vi "HOST_GIPO.vi"() -> ()   [LabVIEW 2018]
uses:
  Program Files (x86)/National Instruments/LabVIEW 2018/examples/Instrument IO/Serial/support/Serial - Settings.ctl
  <instrlib>/niDCPower/nidcpower.llb/niDCPower Measurement Type.ctl
  <vilib>/Instr/_visa.llb/VISA Configure Serial Port (Instr).vi
panel:
  out "CPTE_0":bool
  in  "Запись":bool
  in  "Инициализация":string[](array[string])=["QUITE 0", "INT 0", "OUTP 0", "PAR 0", "PAR:DEL 0", "CH:1:THR 50", "CH:2:THR 50", "CH:3:THR 50", "CH:4:THR 50"]
  in  "Команды":string="INT [1,0,?] - Enabled/Disabled/Get Interrupt\nQUITE [1,0,?] - Enabled/Disabled/Get QuiteMode\nOUTP [1,0,?] - On/Off/Get Output\nRESU - Block parry, on output and unblock parry\nRESU:DEL - Delay in ms of block parry\nRESU:AUTO [1,0,?] - Auto resume after parry\nRESU:AUTO:DEL - Delay in ms of Auto resume\nMON [1,0,?] - Enabled/Disabled/Get Monitor\nMON:DEL [0-1000,?] - Set/Get Monitor Delay in ms of Monitor\nPAR [1,0,?] - Enabled/Disabled/Get Parry\nPAR:DEL [0-1000,?] - Set/Get Parry Delay in ms of Parry\nCH:i:MEAS:CURR? - Measure current in channel [i]\nCH:i:MAX:CURR? - Get max current in channel [i], and clear value\nCH:i:THR [20-3330,?] - Set/Get Threshold current in mA in channel [i] of SEL Event\nCH:i:STAT? - Get State of channel [i]\nUse number 0 for alternate channel, and Threshold from [1-1666] mA\nCHSSTAT? - Get State channels\nCHSEXST? - Get Exist channels\nCNT? - Get count SEL\nCNT:CLR - Clear count SEL\nWIRECLOCK [100000,400000] - set I2C clock\nTEST - Self test ADC + DAC + Triggers"
  in  "Ручной(Т)/Авто":bool
  in  "Log":string="Ниже представлен лог общения с СПТЭ:\nParry Scheme initialized.v2.9.2 + Alt Channel\nSend <HELP> to see commands.\nNow set Ipar = 333 mA (Upar = 0.5 V, Upar_alt = 3.0 V)\nExist channels\nCh1 : 1\nCh2 : 1\nCh3 : 1\nCh4 : 1\nCh_alt0 : 0\nREADY\nQUITE Off\nINT Off\nOUTP Off\nPAR Off\nPAR:DEL: 0 ms\nIn ch1 (DAC 0xC) set Ipar = 20 mA (0.030 V)\nIn ch2 (DAC 0xD) set Ipar = 20 mA (0.030 V)\nIn ch3 (DAC 0xE) set Ipar = 20 mA (0.030 V)\nIn ch4 (DAC 0x8) set Ipar = 20 mA (0.030 V)\ninvalid String, send <HELP> for see commands\nDEBUG:ttyData=\nlength=0\n0x00 0x00 0x00 0x00 0x00 0x00 \n"
  out "CPTE":i32
  out "CPTE":bool
  out "CPTE =":string
  in  "Опрос":bool
  in  "Питание матрицы":bool
  in  "Emt(T)/Enter(F)":bool
  out "Номер образца":string="0"
  in  "SEL":path=path "C:/LabView_PRJ/22.099_GIPO/SEL"
  in  "V_2/GIPO":refnum<k15>="PXI1Slot4" caption="instrument handle"
  in  "V_18/V_65":refnum<k15>="PXI1Slot3" caption="instrument handle"
  in  "V_5/V_55":refnum<k15>="PXI1Slot2" caption="instrument handle"
  out "GIPO Chart":dbl(graph)=0.0015269744355577005 caption="Waveform Chart 5"
  out "GIPO_cur, A":dbl caption="measurement" format="%_6g"
  in  "GIPO_curlim, A":dbl=1.0 caption="current limit" format="%_6p"
  in  "GIPO, V":dbl=16.0 caption="voltage level" format="%_6p"
  out "V_2 Chart":dbl(graph)=0.012083984740959104 caption="Waveform Chart 5"
  out "V_2_cur, A":dbl caption="measurement" format="%_6g"
  in  "V_2_curlim, A":dbl=0.1 caption="current limit" format="%_6p"
  in  "V_2, V":dbl=2.048 caption="voltage level" format="%_6p"
  in  "Питание":bool
  out "V_65 Chart":dbl(graph)=0.002248520443690256
  out "V_65_cur, A":dbl caption="measurement" format="%_6g"
  in  "V_65, V":dbl=6.5 caption="voltage level" format="%_6p"
  in  "V_65_curlim, A":dbl=0.1 caption="current limit" format="%_6p"
  out "V_5 Chart":dbl(graph)=0.10501062604189042 caption="Waveform Chart 5"
  out "V_18 Chart":dbl(graph)=0.06950688300254347
  out "V_55 Chart":dbl(graph)=0.0003386853255381902
  out "V_18_cur, A":dbl caption="measurement" format="%_6g"
  in  "V_18_curlim, A":dbl=0.1 caption="current limit" format="%_6p"
  in  "V_18, V":dbl=1.8 caption="voltage level" format="%_6p"
  in  "V_55, V":dbl=5.5 caption="voltage level" format="%_6p"
  out "V_55_cur, A":dbl caption="measurement" format="%_6g"
  out "V_5_cur, A":dbl caption="measurement" format="%_6g"
  in  "V_55_curlim, A":dbl=0.1 caption="current limit" format="%_6p"
  in  "V_5_curlim, A":dbl=0.1 caption="current limit" format="%_6p"
  in  "V_5, V":dbl=5.0 caption="voltage level" format="%_6p"
  in  "Стоп":bool
  in  "Период, мс":u32=1
  out "V_2":bool
  out "V_2":i32
  in  "V_2_selcur":dbl=0.01 caption="current limit" format="%_6p"
  out "V_65":bool
  out "V_65":i32
  in  "V_65_selcur":dbl=0.01 caption="current limit" format="%_6p"
  out "V_18":bool
  out "V_18":i32
  out "V_55":bool
  out "V_55":i32
  out "V_5":bool
  out "V_5":i32
  in  "V_18_selcur":dbl=0.01 caption="current limit" format="%_6p"
  in  "V_55_selcur":dbl=0.01 caption="current limit" format="%_6p"
  in  "V_5_selcur":dbl=0.01 caption="current limit" format="%_6p"
  out "SEL":bool
  in  "SIM_SEL":bool
  out "GIPO":bool
  out "GIPO":i32
  in  "GIPO_selcur":dbl=0.95 caption="current limit" format="%_6p"
  in  "Питание оснастки":bool
  in  "Command":string="PAR 0"
  in  "Serial Settings":T1={"baud rate"=115200, "data bits"=8, "parity"=enum."None", "stop bits"=10, "flow control"=0} {"flow control" items=["None"=0, "XON/XOFF"=1, "RTS/CTS"=2, "DTR/DSR"=4]; "stop bits" items=["1.0"=10, "1.5"=15, "2.0"=20]; "data bits" min=5 max=8 step=1; "baud rate" items=["75"=75, "110"=110, "134"=134, "150"=150, "300"=300, "600"=600, "1200"=1200, "1800"=1800, "2400"=2400, "4800"=4800, "7200"=7200, "9600"=9600, "14400"=14400, "19200"=19200, "28800"=28800, "38400"=38400, "56000"=56000, "57600"=57600, "115200"=115200, "128000"=128000, "230400"=230400]}
  in  "VISA resource name":refnum<visa-resource-name>="COM4"
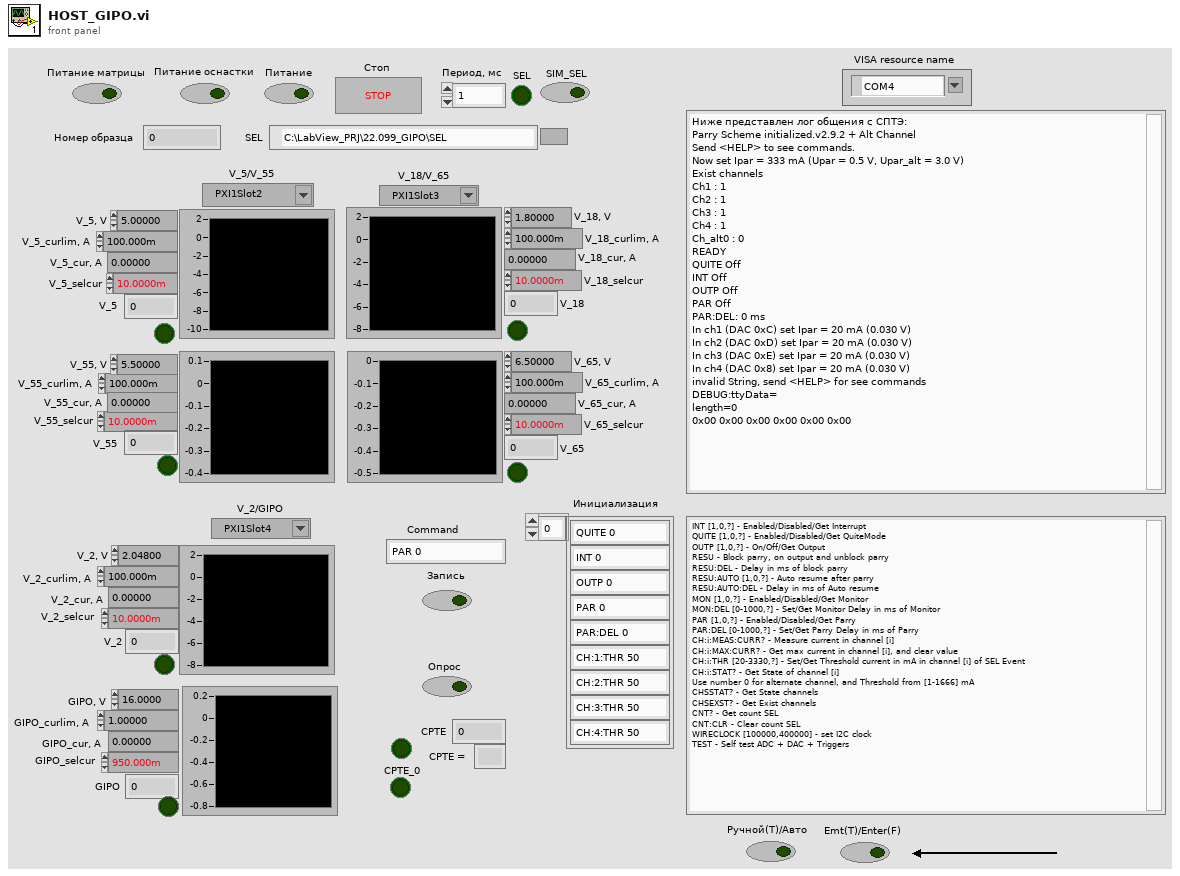
[diagram p1: front panel]
types:
  T1 = typedef "Serial - Settings.ctl" = cluster{"baud rate":u32, "data bits":u16, "parity":enum16{"None", "Odd", "Even", "Mark", "Space"}, "stop bits":u16, "flow control":u16}
  T2 = enum16{"open", "replace", "create", "open or create", "replace or create", "replace or create with confirmation"}
  T3 = enum16{"Native", "Native Command Line", "UNIX", "Macintosh", "DOS"}
  T4 = typedef "niDCPower Measurement Type.ctl" = i32
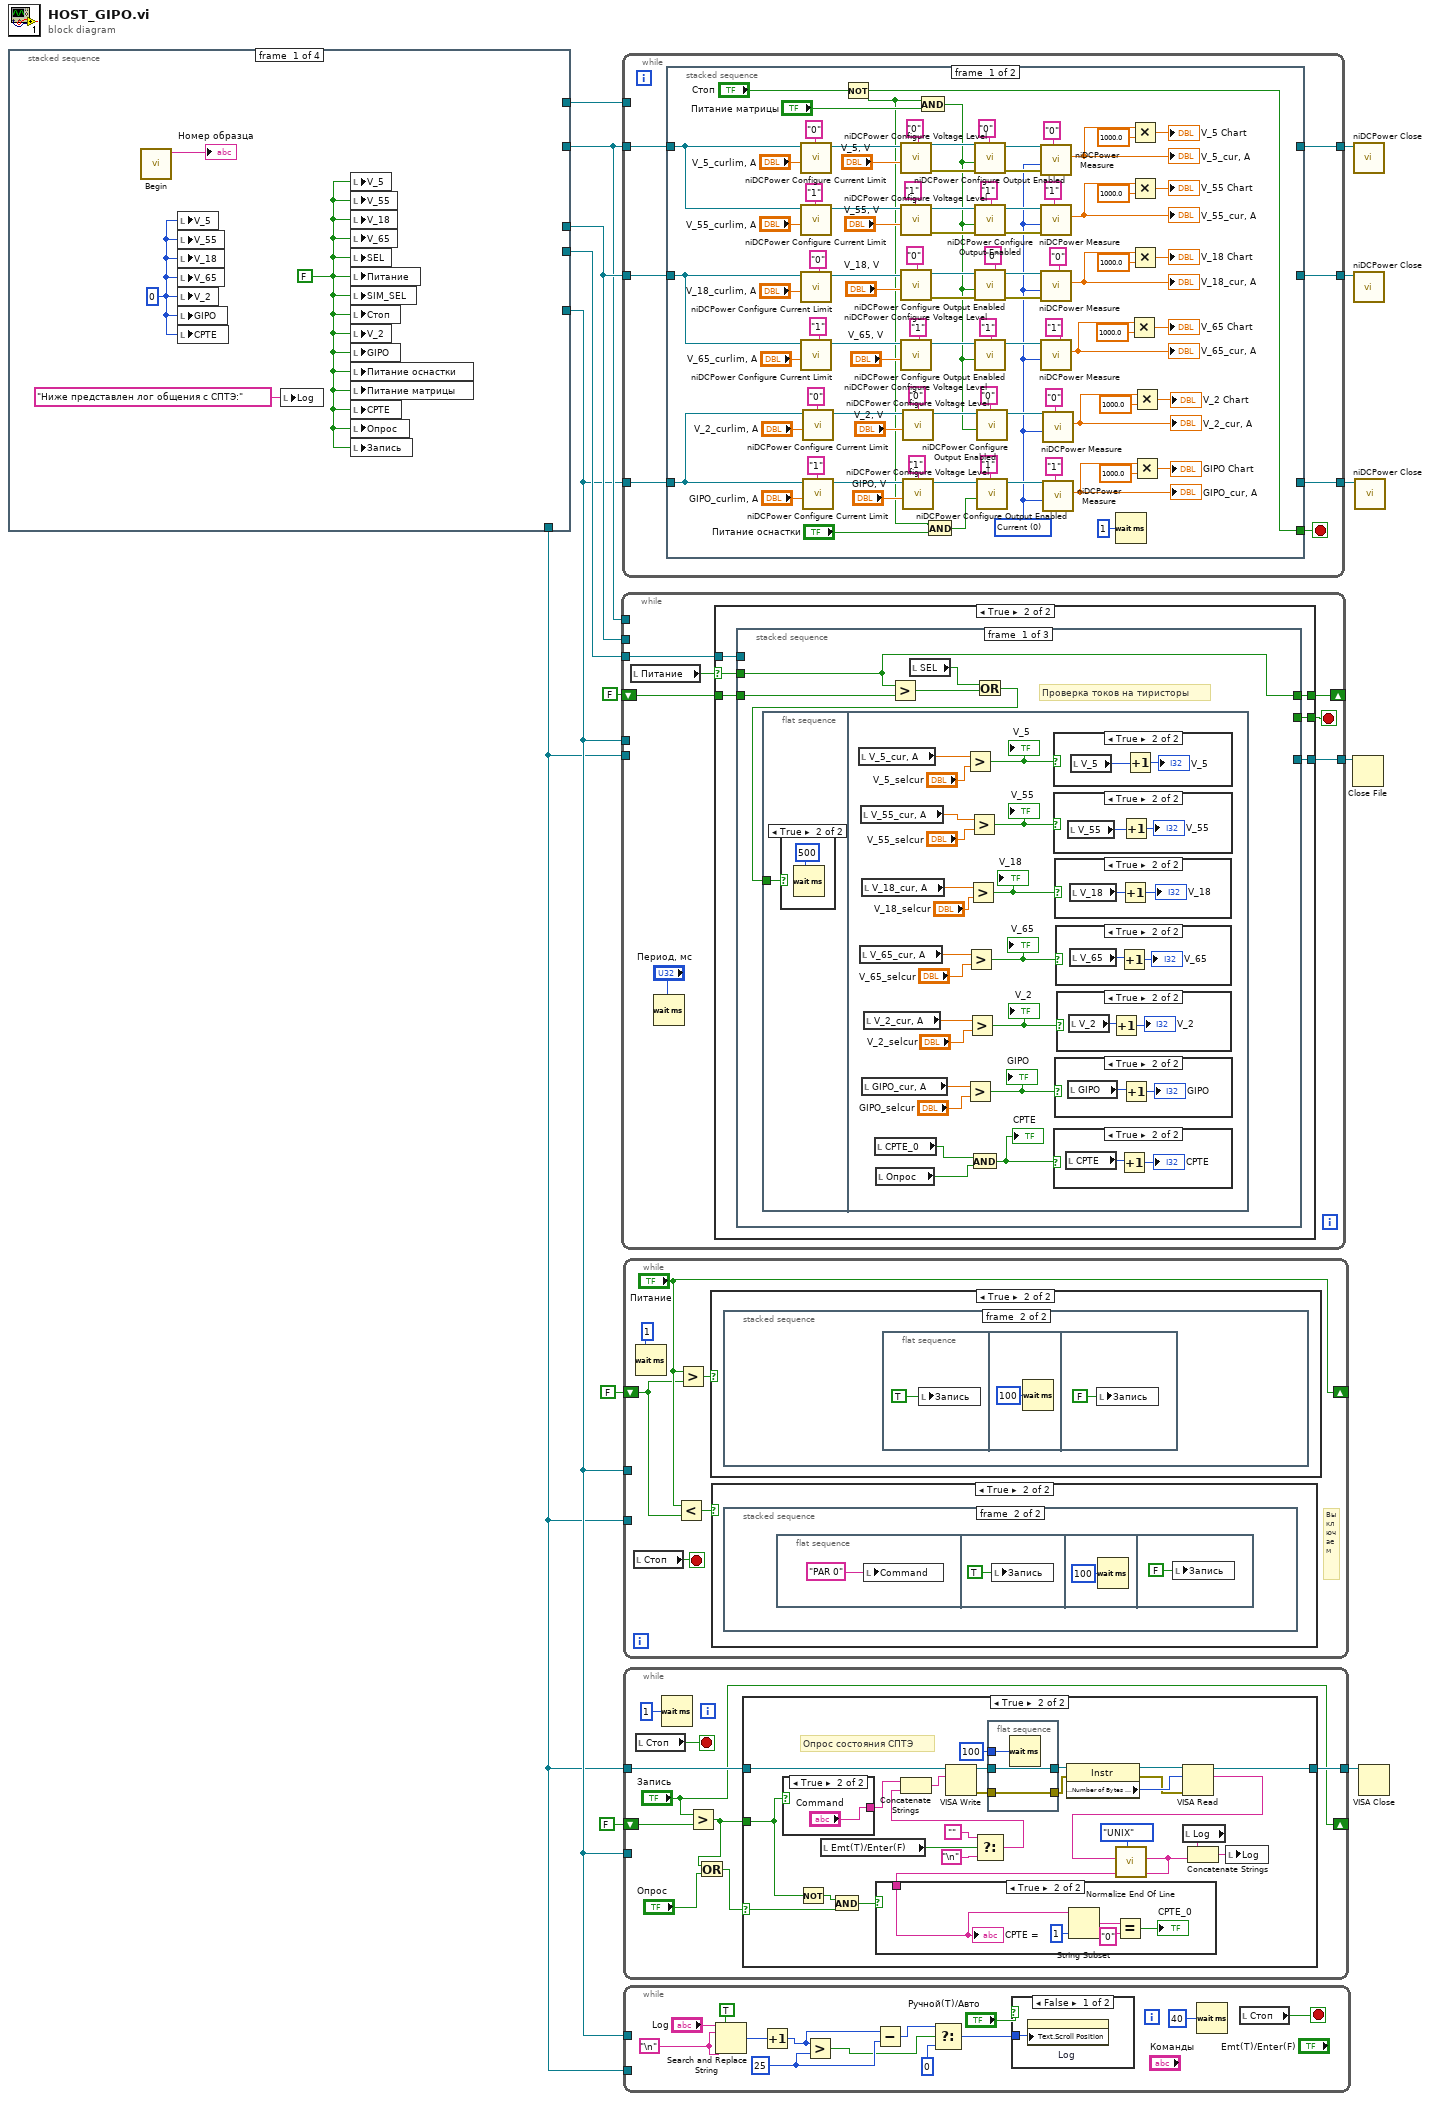
[diagram p0: block diagram]
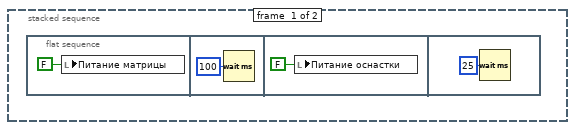
[diagram p3: hidden frame]
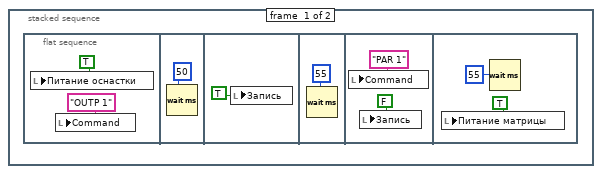
[diagram p5: hidden frame]
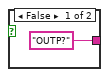
[diagram p8: hidden frame]
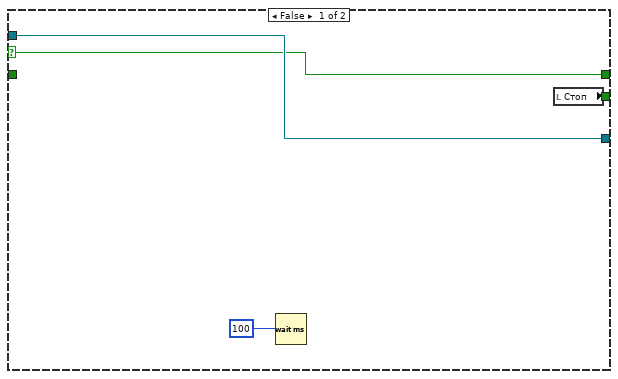
[diagram p10: hidden frame]
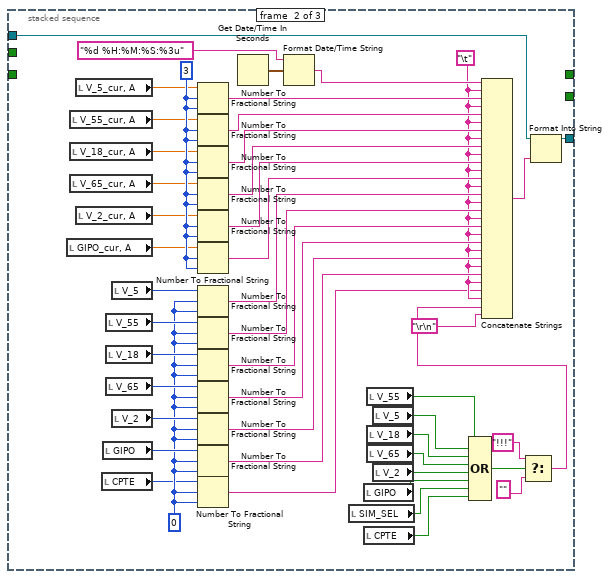
[diagram p19: hidden frame]
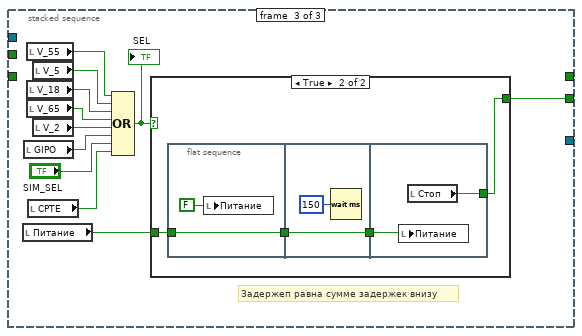
[diagram p20: hidden frame]
diagram:
  n1 = stacked-sequence {
    tunnel: [_ _ w67 _] -> w11
    tunnel: [_ _ w66 _] -> w10
    tunnel: [_ w36 _ _] -> w13
    tunnel: [_ _ w60 _] -> w5
    tunnel: [_ _ _ w85] -> w6
    tunnel: [_ _ _ w85] -> w4
    frame #0 {
      w17 = 0
      w16 = FALSE
      n2 = call "Begin.vi"() -> ("Номер образца 2"=→"Номер образца":string)  [unwired: 11 in]
      n3 = local write "V_5"(w17) -> ()
      n4 = local write "V_55"(w17) -> ()
      n5 = local write "V_18"(w17) -> ()
      n6 = local write "V_65"(w17) -> ()
      n7 = local write "V_2"(w17) -> ()
      n8 = local write "GIPO"(w17) -> ()
      n9 = local write "CPTE"(w17) -> ()
      n10 = local write "Log"("Ниже представлен лог общения с СПТЭ:") -> ()
      n11 = local write "V_5"(w16) -> ()
      n12 = local write "V_55"(w16) -> ()
      n13 = local write "V_18"(w16) -> ()
      n14 = local write "V_65"(w16) -> ()
      n15 = local write "SEL"(w16) -> ()
      n16 = local write "Питание"(w16) -> ()
      n17 = local write "SIM_SEL"(w16) -> ()
      n18 = local write "Стоп"(w16) -> ()
      n19 = local write "V_2"(w16) -> ()
      n20 = local write "GIPO"(w16) -> ()
      n21 = local write "Питание оснастки"(w16) -> ()
      n22 = local write "Питание матрицы"(w16) -> ()
      n23 = local write "CPTE"(w16) -> ()
      n24 = local write "Опрос"(w16) -> ()
      n25 = local write "Запись"(w16) -> ()
    }
    frame #1 {
      w21 = "\t"
      # "Инициализаци первой строки лога по токам"
      n26 = local read "Номер образца"() -> (w48:string)
      n27 = Build Path(base path="SEL", name or relative path=w48) -> (appended path=w50:path)
      n28 = Get Date/Time In Seconds() -> (seconds since 1Jan1904=w43:timestamp)
      n29 = call <vilib>:"Check if File or Folder Exists.vi"("path"=w50) -> ("file or folder exists?"=w51:bool, "dup path"=w52:path)  [unwired: 8 in, 1 out]
      n30 = Format Date/Time String(time format string (%c)="%d %H.%M.%S", seconds (now)=w43) -> (date/time string=w40:string)  [unwired: 1 in]
      n31 = case shown="False" w51 {
        tunnel: w52 -> [w58 w59]
        tunnel: [w57 w59] -> w35
        frame False {
          n32 = Create Folder(path (use dialog)=w58) -> (created path=w57:path)  [unwired: 2 in, 2 out]
        }
        frame True {
        }
      }
      n33 = Concatenate Strings(w40, ".xls" ("string")) -> (w38:string)
      n34 = Build Path(base path=w35, name or relative path=w38) -> (appended path=w41:path)
      n35 = Open/Create/Replace File(file path (use dialog)=w41, operation (0:open)=T2."open or create", access (0:read/write)=enum16{"read/write", "read-only", "write-only"}."read/write") -> (refnum out=w44:refnum<file>)  [unwired: 3 in, 2 out]
      n36 = case shown="True" TRUE {
        tunnel: w44 -> [w53 w56]
        tunnel: [w53 w54] -> w37
        frame False {
        }
        frame True {
          n37 = Set File Position(refnum=w56, from (0:start)=enum16{"start", "end", "current"}."end") -> (refnum out=w54:refnum<file>)  [unwired: 2 in, 1 out]
        }
      }
      n38 = Format Into String(initial string=w37, "Time" ("input 1"), w21, "V_5_cur " ("input 1"), w21, "V_55_cur " ("input 1"), w21, "V_18_cur " ("input 1"), w21, "V_65_cur " ("input 1"), w21, "V_2_cur " ("input 1"), w21, "GIPO_cur " ("input 1"), w21, "V_5" ("input 1"), w21, "V_55" ("input 1"), w21, "V_18" ("input 1"), w21, "V_65" ("input 1"), w21, "V_2" ("input 1"), w21, "GIPO" ("input 1"), w21, "CPTE" ("input 1"), "\r\n") -> (resulting string=w36:refnum<file>)  [unwired: 2 in, 1 out]
    }
    frame #2 {
      n39 = call <instrlib>:"niDCPower Initialize.vi"("resource name"="V_2/GIPO") -> ("error out"=w63:errorcluster, "instrument handle out"=w62:refnum<k15>)  [unwired: 3 in, 6 out]
      n40 = call <instrlib>:"niDCPower Initialize.vi"("resource name"="V_5/V_55") -> ("error out"=w74:errorcluster, "instrument handle out"=w76:refnum<k15>)  [unwired: 3 in, 6 out]
      n41 = call <instrlib>:"niDCPower Initialize.vi"("resource name"="V_18/V_65") -> ("error out"=w75:errorcluster, "instrument handle out"=w77:refnum<k15>)  [unwired: 3 in, 6 out]
      n42 = call <instrlib>:"niDCPower Configure Voltage Level.vi"("error in (no error)"=w74, "voltage level"=0.0, "channel name"="0,1", "instrument handle"=w76) -> ("instrument handle out"=w66:refnum<k15>)  [unwired: 6 in, 1 out]
      n43 = call <instrlib>:"niDCPower Configure Voltage Level.vi"("error in (no error)"=w75, "voltage level"=0.0, "channel name"="0,1", "instrument handle"=w77) -> ("instrument handle out"=w67:refnum<k15>)  [unwired: 6 in, 1 out]
      n44 = call <instrlib>:"niDCPower Configure Voltage Level.vi"("error in (no error)"=w63, "voltage level"=0.0, "channel name"="0,1", "instrument handle"=w62) -> ("instrument handle out"=w60:refnum<k15>)  [unwired: 6 in, 1 out]
    }
    frame #3 {
      n45 = Unbundle By Name("Serial Settings") -> ("baud rate"=w98:u32, "data bits"=w97:u16, "parity"=w96:enum16{"None", "Odd", "Even", "Mark", "Space"}, "stop bits"=w95:u16, "flow control"=w94:u16)
      n46 = for {
        tunnel: "Инициализация" -> [w108] mode=indexing
        tunnel: w87 -> [w111]
        tunnel: [w109] -> w86
        n47 = local read "Emt(T)/Enter(F)"() -> (w106:bool)
        n48 = Select(t="", s=w106, f="\n") -> (s? t:f=w103:string)
        n49 = Concatenate Strings(w108, w103) -> (w107:string)
        n50 = VISA Write(VISA resource name=w111, write buffer=w107) -> (VISA resource name out=w110:refnum<visa-resource-name>)  [unwired: 1 in, 2 out]
        n51 = flat-sequence {
          tunnel: [w113] -> w109
          tunnel: w110 -> [w113]
          frame #0 {
            n52 = Wait (ms)(milliseconds to wait=u32 100) -> ()  [unwired: 1 out]
          }
        }
      }
      n53 = property class="Instr"(reference=w86) -> (reference out=w91:refnum<visa-resource-name>, error out=w90:errorcluster, "Serial Settings:Number of Bytes at Serial Port"=w89:u32)  [unwired: 1 in]
      n54 = VISA Read(VISA resource name=w91, byte count=w89, error in (no error)=w90) -> (VISA resource name out=w85:refnum<visa-resource-name>, read buffer=w83:string)  [unwired: 2 out]
      n55 = call-poly "VISA Configure Serial Port"("VISA resource name"="VISA resource name", "termination char\n(0xA = '\\n' = LF)"=u8 10 ("termination char\n(0xA = '\\n' = LF)"), "Enable Termination\nChar (T)"=FALSE ("Enable Termination\nChar (T)"), "baud rate (9600)"=w98, "data bits (8)"=w97, "parity (0:none)"=w96, "stop bits (10: 1 bit)"=w95, "flow control (0:none)"=w94) -> ("VISA resource name out"=w88:refnum<visa-resource-name>)  [unwired: 2 in, 5 out]
      n56 = call <vilib>:"Normalize End Of Line.vi"("end of line (Native)"=T3."UNIX", "string in"=w83) -> ("string out"=w82:string)  [unwired: 6 in]
      n57 = flat-sequence {
        tunnel: w88 -> [w101]
        tunnel: [w101] -> w87
        frame #0 {
          n58 = Wait (ms)(milliseconds to wait=u32 2000) -> ()  [unwired: 1 out]
        }
      }
      n59 = local read "Log"() -> (w80:string)
      n60 = Concatenate Strings(w80, "\n", w82) -> (w84:string)
      n61 = local write "Log"(w84) -> ()
    }
  }
  n62 = while {
    shift-right: [w114] -> _
    shift-left: FALSE -> [w120]
    tunnel: w13 -> [w119]
    tunnel: [w117] -> w12
    tunnel: w5 -> [_]
    tunnel: w11 -> [_]
    tunnel: w10 -> [_]
    tunnel: w4 -> [_]
    stop <- w118 stop-if-true
    n63 = local read "Питание"() -> (w115:bool)
    n64 = Wait (ms)(milliseconds to wait="Период, мс") -> ()  [unwired: 1 out]
    n65 = case shown="True" w115 {
      selector: w115 -> [w121 w126]
      tunnel: w120 -> [_ w130]
      tunnel: w119 -> [w123 w129]
      tunnel: [w124 w128] -> w118
      tunnel: [w123 w127] -> w117
      tunnel: [w121 w125] -> w114
      frame False {
        n66 = Wait (ms)(milliseconds to wait=u32 100 ("f")) -> ()  [unwired: 1 out]
        n67 = local read "Стоп"() -> (w124:bool)
      }
      frame True {
        n68 = stacked-sequence {
          tunnel: w130 -> [w135 _ _]
          tunnel: w129 -> [_ w210 _]
          tunnel: [_ _ w222] -> w128
          tunnel: [_ w208 _] -> w127
          tunnel: w126 -> [w131 _ _]
          tunnel: [w131 _ _] -> w125
          frame #0 {
            # "Проверка токов на тиристоры"
            n69 = flat-sequence {
              tunnel: w132 -> [w136]
              frame #0 {
                n70 = case shown="True" w136 {
                  frame False {
                  }
                  frame True {
                    n71 = Wait (ms)(milliseconds to wait=u32 500) -> ()  [unwired: 1 out]
                  }
                }
              }
              frame #1 {
                n72 = local read "V_5_cur, A"() -> (w152:dbl)
                n73 = local read "V_65_cur, A"() -> (w149:dbl)
                n74 = local read "V_55_cur, A"() -> (w151:dbl)
                n75 = local read "V_18_cur, A"() -> (w150:dbl)
                n76 = local read "GIPO_cur, A"() -> (w141:dbl)
                n77 = local read "V_2_cur, A"() -> (w144:dbl)
                n78 = local read "CPTE_0"() -> (w139:bool)
                n79 = local read "Опрос"() -> (w138:bool)
                n80 = Greater?(x=w152, y="V_5_selcur") -> (0:w157:bool)
                "V_5" <- w157
                n81 = Greater?(x=w141, y="GIPO_selcur") -> (0:w143:bool)
                "GIPO" <- w143
                n82 = Greater?(x=w149, y="V_65_selcur") -> (0:w148:bool)
                "V_65" <- w148
                n83 = Greater?(x=w144, y="V_2_selcur") -> (0:w145:bool)
                "V_2" <- w145
                n84 = Greater?(x=w150, y="V_18_selcur") -> (0:w153:bool)
                "V_18" <- w153
                n85 = Greater?(x=w151, y="V_55_selcur") -> (0:w155:bool)
                "V_55" <- w155
                n86 = And(x=w139, y=w138) -> (x .and. y?=w140:bool)
                "CPTE" <- w140
                n87 = case shown="True" w157 {
                  frame False {
                  }
                  frame True {
                    n88 = local read "V_5"() -> (w172:i32)
                    n89 = Increment(x=w172) -> (x+1=→"V_5":i32)
                  }
                }
                n90 = case shown="True" w155 {
                  frame False {
                  }
                  frame True {
                    n91 = local read "V_55"() -> (w169:i32)
                    n92 = Increment(x=w169) -> (x+1=→"V_55":i32)
                  }
                }
                n93 = case shown="True" w140 {
                  frame False {
                  }
                  frame True {
                    n94 = local read "CPTE"() -> (w160:i32)
                    n95 = Increment(x=w160) -> (x+1=→"CPTE":i32)
                  }
                }
                n96 = case shown="True" w153 {
                  frame False {
                  }
                  frame True {
                    n97 = local read "V_18"() -> (w168:i32)
                    n98 = Increment(x=w168) -> (x+1=→"V_18":i32)
                  }
                }
                n99 = case shown="True" w143 {
                  frame False {
                  }
                  frame True {
                    n100 = local read "GIPO"() -> (w162:i32)
                    n101 = Increment(x=w162) -> (x+1=→"GIPO":i32)
                  }
                }
                n102 = case shown="True" w148 {
                  frame False {
                  }
                  frame True {
                    n103 = local read "V_65"() -> (w166:i32)
                    n104 = Increment(x=w166) -> (x+1=→"V_65":i32)
                  }
                }
                n105 = case shown="True" w145 {
                  frame False {
                  }
                  frame True {
                    n106 = local read "V_2"() -> (w164:i32)
                    n107 = Increment(x=w164) -> (x+1=→"V_2":i32)
                  }
                }
              }
            }
            n108 = Greater?(x=w131, y=w135) -> (0:w134:bool)
            n109 = local read "SEL"() -> (w133:bool)
            n110 = Or(x=w133, y=w134) -> (x .or. y?=w132:bool)
          }
          frame #1 {
            w178 = i16 0 ("width (-)")
            w207 = i16 3 ("width (-)")
            w179 = "\t"
            n111 = local read "GIPO_cur, A"() -> (w198:dbl)
            n112 = local read "V_55_cur, A"() -> (w202:dbl)
            n113 = local read "V_18_cur, A"() -> (w201:dbl)
            n114 = local read "V_65_cur, A"() -> (w200:dbl)
            n115 = local read "V_5_cur, A"() -> (w203:dbl)
            n116 = local read "V_2_cur, A"() -> (w199:dbl)
            n117 = local read "CPTE"() -> (w177:i32)
            n118 = local read "GIPO"() -> (w188:i32)
            n119 = local read "V_55"() -> (w196:i32)
            n120 = local read "V_18"() -> (w195:i32)
            n121 = local read "V_65"() -> (w194:i32)
            n122 = local read "V_5"() -> (w197:i32)
            n123 = local read "V_2"() -> (w193:i32)
            n124 = Number To Fractional String(number=w203, width (-)=w207, precision (6)=w207) -> (F-format string=w214:string)  [unwired: 1 in]
            n125 = Number To Fractional String(number=w202, width (-)=w207, precision (6)=w207) -> (F-format string=w213:string)  [unwired: 1 in]
            n126 = Number To Fractional String(number=w201, width (-)=w207, precision (6)=w207) -> (F-format string=w212:string)  [unwired: 1 in]
            n127 = Number To Fractional String(number=w200, width (-)=w207, precision (6)=w207) -> (F-format string=w209:string)  [unwired: 1 in]
            n128 = Number To Fractional String(number=w199, width (-)=w207, precision (6)=w207) -> (F-format string=w205:string)  [unwired: 1 in]
            n129 = Number To Fractional String(number=w198, width (-)=w207, precision (6)=w207) -> (F-format string=w204:string)  [unwired: 1 in]
            n130 = Number To Fractional String(number=w197, width (-)=w178, precision (6)=w178) -> (F-format string=w185:string)  [unwired: 1 in]
            n131 = Number To Fractional String(number=w196, width (-)=w178, precision (6)=w178) -> (F-format string=w184:string)  [unwired: 1 in]
            n132 = Number To Fractional String(number=w195, width (-)=w178, precision (6)=w178) -> (F-format string=w183:string)  [unwired: 1 in]
            n133 = Number To Fractional String(number=w194, width (-)=w178, precision (6)=w178) -> (F-format string=w182:string)  [unwired: 1 in]
            n134 = Number To Fractional String(number=w193, width (-)=w178, precision (6)=w178) -> (F-format string=w181:string)  [unwired: 1 in]
            n135 = Number To Fractional String(number=w188, width (-)=w178, precision (6)=w178) -> (F-format string=w180:string)  [unwired: 1 in]
            n136 = Number To Fractional String(number=w177, width (-)=w178, precision (6)=w178) -> (F-format string=w176:string)  [unwired: 1 in]
            n137 = Get Date/Time In Seconds() -> (seconds since 1Jan1904=w220:timestamp)
            n138 = Format Date/Time String(time format string (%c)="%d %H:%M:%S:%3u", seconds (now)=w220) -> (date/time string=w215:string)  [unwired: 1 in]
            n139 = local read "SIM_SEL"() -> (w186:bool)
            n140 = local read "GIPO"() -> (w187:bool)
            n141 = local read "CPTE"() -> (w173:bool)
            n142 = local read "V_55"() -> (w192:bool)
            n143 = local read "V_18"() -> (w190:bool)
            n144 = local read "V_65"() -> (w189:bool)
            n145 = local read "V_5"() -> (w191:bool)
            n146 = local read "V_2"() -> (w206:bool)
            n147 = Compound Arithmetic op=OR(w192, w191, w190, w189, w206, w187, w186, w173) -> (w211:bool)
            n148 = Select(t="!!!", s=w211, f="") -> (s? t:f=w175:string)
            n149 = Concatenate Strings(w215, w179, w214, w179, w213, w179, w212, w179, w209, w179, w205, w179, w204, w179, w185, w179, w184, w179, w183, w179, w182, w179, w181, w179, w180, w179, w176, w179, w175, "\r\n") -> (w219:string)
            n150 = Format Into String(initial string=w210, w219) -> (resulting string=w208:refnum<file>)  [unwired: 2 in, 1 out]
          }
          frame #2 {
            # "Задержеп равна сумме задержек внизу"
            n151 = local read "Питание"() -> (w221:bool)
            n152 = local read "GIPO"() -> (w225:bool)
            n153 = local read "V_55"() -> (w229:bool)
            n154 = local read "V_18"() -> (w227:bool)
            n155 = local read "V_65"() -> (w226:bool)
            n156 = local read "CPTE"() -> (w223:bool)
            n157 = local read "V_5"() -> (w228:bool)
            n158 = local read "V_2"() -> (w231:bool)
            n159 = Compound Arithmetic op=OR(w229, w228, w227, w226, w231, w225, "SIM_SEL", w223) -> (w230:bool)
            "SEL" <- w230
            n160 = case shown="True" w230 {
              tunnel: [w232 w233] -> w222
              tunnel: w221 -> [_ w234]
              frame False {
                n161 = local read "Стоп"() -> (w232:bool)
              }
              frame True {
                n162 = flat-sequence {
                  tunnel: [w237] -> w235
                  tunnel: w234 -> [w237]
                  tunnel: [w239] -> w236
                  tunnel: w235 -> [w239]
                  tunnel: w236 -> [w242]
                  tunnel: [w241] -> w233
                  frame #0 {
                    n163 = local write "Питание"(FALSE ("Питание")) -> ()
                  }
                  frame #1 {
                    n164 = Wait (ms)(milliseconds to wait=u32 150) -> ()  [unwired: 1 out]
                  }
                  frame #2 {
                    n165 = local write "Питание"(w242) -> ()
                    n166 = local read "Стоп"() -> (w241:bool)
                  }
                }
              }
            }
          }
        }
      }
    }
  }
  n167 = while {
    tunnel: w10 -> [w249]
    tunnel: w5 -> [w247]
    tunnel: w11 -> [w248]
    tunnel: [w246] -> w9
    tunnel: [w245] -> w8
    tunnel: [w244] -> w7
    tunnel: w6 -> [_]
    stop <- w243 stop-if-true
    n168 = stacked-sequence {
      tunnel: w247 -> [w258 w339]
      tunnel: w248 -> [w257 w340]
      tunnel: w249 -> [w256 w341]
      tunnel: [_ w341] -> w246
      tunnel: [_ w340] -> w245
      tunnel: [_ w339] -> w244
      tunnel: ["Стоп" _] -> w243
      frame #0 {
        w259 = T4 0 items=["Current", "Voltage"] ("measurement type")
        n169 = call <instrlib>:"niDCPower Configure Current Limit.vi"("current limit"="V_5_curlim, A", "channel name"="0", "instrument handle"=w256) -> ("instrument handle out"=w327:refnum<k15>)  [unwired: 7 in, 1 out]
        n170 = call <instrlib>:"niDCPower Configure Current Limit.vi"("current limit"="V_55_curlim, A", "channel name"="1", "instrument handle"=w256) -> ("instrument handle out"=w328:refnum<k15>)  [unwired: 7 in, 1 out]
        n171 = call <instrlib>:"niDCPower Configure Current Limit.vi"("current limit"="V_18_curlim, A", "channel name"="0", "instrument handle"=w257) -> ("instrument handle out"=w310:refnum<k15>)  [unwired: 7 in, 1 out]
        n172 = call <instrlib>:"niDCPower Configure Current Limit.vi"("current limit"="V_65_curlim, A", "channel name"="1", "instrument handle"=w257) -> ("instrument handle out"=w290:refnum<k15>)  [unwired: 7 in, 1 out]
        n173 = call <instrlib>:"niDCPower Configure Current Limit.vi"("current limit"="V_2_curlim, A", "channel name"="0", "instrument handle"=w258) -> ("instrument handle out"=w281:refnum<k15>)  [unwired: 7 in, 1 out]
        n174 = call <instrlib>:"niDCPower Configure Current Limit.vi"("current limit"="GIPO_curlim, A", "channel name"="1", "instrument handle"=w258) -> ("instrument handle out"=w262:refnum<k15>)  [unwired: 7 in, 1 out]
        n175 = Not(x="Стоп") -> (.not. x?=w250:bool)
        n176 = call <instrlib>:"niDCPower Configure Voltage Level.vi"("voltage level"="V_5, V", "channel name"="0", "instrument handle"=w327) -> ("error out"=w320:errorcluster, "instrument handle out"=w323:refnum<k15>)  [unwired: 7 in]
        n177 = call <instrlib>:"niDCPower Configure Voltage Level.vi"("voltage level"="V_55, V", "channel name"="1", "instrument handle"=w328) -> ("error out"=w321:errorcluster, "instrument handle out"=w322:refnum<k15>)  [unwired: 7 in]
        n178 = call <instrlib>:"niDCPower Configure Voltage Level.vi"("voltage level"="V_18, V", "channel name"="0", "instrument handle"=w310) -> ("error out"=w314:errorcluster, "instrument handle out"=w315:refnum<k15>)  [unwired: 7 in]
        n179 = call <instrlib>:"niDCPower Configure Voltage Level.vi"("voltage level"="V_65, V", "channel name"="1", "instrument handle"=w290) -> ("instrument handle out"=w288:refnum<k15>)  [unwired: 7 in, 1 out]
        n180 = call <instrlib>:"niDCPower Configure Voltage Level.vi"("voltage level"="V_2, V", "channel name"="0", "instrument handle"=w281) -> ("instrument handle out"=w280:refnum<k15>)  [unwired: 7 in, 1 out]
        n181 = call <instrlib>:"niDCPower Configure Voltage Level.vi"("voltage level"="GIPO, V", "channel name"="1", "instrument handle"=w262) -> ("instrument handle out"=w263:refnum<k15>)  [unwired: 7 in, 1 out]
        n182 = And(x=w250, y="Питание матрицы") -> (x .and. y?=w255:bool)
        n183 = And(x=w250, y="Питание оснастки") -> (x .and. y?=w251:bool)
        n184 = call <instrlib>:"niDCPower Configure Output Enabled.vi"("error in (no error)"=w320, "output enabled"=w255, "channel name"="0", "instrument handle"=w323) -> ("error out"=w332:errorcluster, "instrument handle out"=w331:refnum<k15>)  [unwired: 6 in]
        n185 = call <instrlib>:"niDCPower Configure Output Enabled.vi"("error in (no error)"=w321, "output enabled"=w255, "channel name"="1", "instrument handle"=w322) -> ("error out"=w333:errorcluster, "instrument handle out"=w334:refnum<k15>)  [unwired: 6 in]
        n186 = call <instrlib>:"niDCPower Configure Output Enabled.vi"("error in (no error)"=w314, "output enabled"=w255, "channel name"="0", "instrument handle"=w315) -> ("error out"=w306:errorcluster, "instrument handle out"=w307:refnum<k15>)  [unwired: 6 in]
        n187 = call <instrlib>:"niDCPower Configure Output Enabled.vi"("output enabled"=w255, "channel name"="1", "instrument handle"=w288) -> ("instrument handle out"=w286:refnum<k15>)  [unwired: 7 in, 1 out]
        n188 = call <instrlib>:"niDCPower Configure Output Enabled.vi"("output enabled"=w255, "channel name"="0", "instrument handle"=w280) -> ("instrument handle out"=w279:refnum<k15>)  [unwired: 7 in, 1 out]
        n189 = call <instrlib>:"niDCPower Configure Output Enabled.vi"("output enabled"=w251, "channel name"="1", "instrument handle"=w263) -> ("instrument handle out"=w264:refnum<k15>)  [unwired: 7 in, 1 out]
        n190 = call <instrlib>:"niDCPower Measure.vi"("error in (no error)"=w332, "measurement type"=w259, "channel name"="0", "instrument handle"=w331) -> ("measurement"=w299:dbl)  [unwired: 5 in, 2 out]
        "V_5_cur, A" <- w299
        n191 = call <instrlib>:"niDCPower Measure.vi"("error in (no error)"=w333, "measurement type"=w259, "channel name"="1", "instrument handle"=w334) -> ("measurement"=w302:dbl)  [unwired: 5 in, 2 out]
        "V_55_cur, A" <- w302
        n192 = call <instrlib>:"niDCPower Measure.vi"("error in (no error)"=w306, "measurement type"=w259, "channel name"="0", "instrument handle"=w307) -> ("measurement"=w300:dbl)  [unwired: 5 in, 2 out]
        "V_18_cur, A" <- w300
        n193 = call <instrlib>:"niDCPower Measure.vi"("measurement type"=w259, "channel name"="1", "instrument handle"=w286) -> ("measurement"=w284:dbl)  [unwired: 6 in, 2 out]
        "V_65_cur, A" <- w284
        n194 = call <instrlib>:"niDCPower Measure.vi"("measurement type"=w259, "channel name"="0", "instrument handle"=w279) -> ("measurement"=w278:dbl)  [unwired: 6 in, 2 out]
        "V_2_cur, A" <- w278
        n195 = call <instrlib>:"niDCPower Measure.vi"("measurement type"=w259, "channel name"="1", "instrument handle"=w264) -> ("measurement"=w265:dbl)  [unwired: 6 in, 2 out]
        "GIPO_cur, A" <- w265
        n196 = Wait (ms)(milliseconds to wait=u32 1) -> ()  [unwired: 1 out]
        n197 = Multiply(x=w284, y=1000.0) -> (x*y=→"V_65 Chart":dbl)
        n198 = Multiply(x=w299, y=1000.0) -> (x*y=→"V_5 Chart":dbl)
        n199 = Multiply(x=w302, y=1000.0) -> (x*y=→"V_55 Chart":dbl)
        n200 = Multiply(x=w300, y=1000.0) -> (x*y=→"V_18 Chart":dbl)
        n201 = Multiply(x=w278, y=1000.0) -> (x*y=→"V_2 Chart":dbl)
        n202 = Multiply(x=w265, y=1000.0) -> (x*y=→"GIPO Chart":dbl)
      }
      frame #1 {
      }
    }
  }
  n203 = while {
    tunnel: w5 -> [_]
    tunnel: w4 -> [_]
    shift-right: ["Питание"] -> _
    shift-left: FALSE ("Питание") -> [w344]
    stop <- w347 stop-if-true
    # "Выключаем"
    n204 = local read "Стоп"() -> (w347:bool)
    n205 = Wait (ms)(milliseconds to wait=u32 1) -> ()  [unwired: 1 out]
    n206 = Less?(x="Питание", y=w344) -> (x < y?=w342:bool)
    n207 = Greater?(x="Питание", y=w344) -> (0:w343:bool)
    n208 = case shown="True" w343 {
      frame False {
      }
      frame True {
        n209 = stacked-sequence {
          frame #0 {
            n210 = flat-sequence {
              frame #0 {
                n211 = local write "Питание оснастки"(TRUE ("Питание оснастки")) -> ()
                n212 = local write "Command"("OUTP 1" ("Command")) -> ()
              }
              frame #1 {
                n213 = Wait (ms)(milliseconds to wait=u32 50) -> ()  [unwired: 1 out]
              }
              frame #2 {
                n214 = local write "Запись"(TRUE ("Запись")) -> ()
              }
              frame #3 {
                n215 = Wait (ms)(milliseconds to wait=u32 55) -> ()  [unwired: 1 out]
              }
              frame #4 {
                n216 = local write "Command"("PAR 1" ("Command")) -> ()
                n217 = local write "Запись"(FALSE ("Запись")) -> ()
              }
              frame #5 {
                n218 = local write "Питание матрицы"(TRUE ("Питание матрицы")) -> ()
                n219 = Wait (ms)(milliseconds to wait=u32 55) -> ()  [unwired: 1 out]
              }
            }
          }
          frame #1 {
            n220 = flat-sequence {
              frame #0 {
                n221 = local write "Запись"(TRUE ("Запись")) -> ()
              }
              frame #1 {
                n222 = Wait (ms)(milliseconds to wait=u32 100) -> ()  [unwired: 1 out]
              }
              frame #2 {
                n223 = local write "Запись"(FALSE ("Запись")) -> ()
              }
            }
          }
        }
      }
    }
    n224 = case shown="True" w342 {
      frame False {
      }
      frame True {
        n225 = stacked-sequence {
          frame #0 {
            n226 = flat-sequence {
              frame #0 {
                n227 = local write "Питание матрицы"(FALSE ("Питание матрицы")) -> ()
              }
              frame #1 {
                n228 = Wait (ms)(milliseconds to wait=u32 100) -> ()  [unwired: 1 out]
              }
              frame #2 {
                n229 = local write "Питание оснастки"(FALSE ("Питание оснастки")) -> ()
              }
              frame #3 {
                n230 = Wait (ms)(milliseconds to wait=u32 25) -> ()  [unwired: 1 out]
              }
            }
          }
          frame #1 {
            n231 = flat-sequence {
              frame #0 {
                n232 = local write "Command"("PAR 0" ("Command")) -> ()
              }
              frame #1 {
                n233 = local write "Запись"(TRUE ("Запись")) -> ()
              }
              frame #2 {
                n234 = Wait (ms)(milliseconds to wait=u32 100) -> ()  [unwired: 1 out]
              }
              frame #3 {
                n235 = local write "Запись"(FALSE ("Запись")) -> ()
              }
            }
          }
        }
      }
    }
  }
  n236 = while {
    tunnel: [w376] -> w2
    tunnel: w5 -> [_]
    tunnel: w4 -> [w374]
    shift-right: ["Запись"] -> _
    shift-left: FALSE ("Запись") -> [w372]
    stop <- w373 stop-if-true
    n237 = local read "Стоп"() -> (w373:bool)
    n238 = Wait (ms)(milliseconds to wait=u32 1) -> ()  [unwired: 1 out]
    n239 = Greater?(x="Запись", y=w372) -> (0:w368:bool)
    n240 = Or(x=w368, y="Опрос") -> (x .or. y?=w369:bool)
    n241 = case shown="True" w369 {
      selector: w369 -> [_ w400]
      tunnel: [w377 w402] -> w376
      tunnel: w374 -> [w377 w401]
      tunnel: w368 -> [_ w378]
      frame False {
      }
      frame True {
        # "Опрос состояния СПТЭ"
        n242 = case shown="True" w378 {
          tunnel: ["OUTP?" "Command"] -> w392
          frame False {
          }
          frame True {
          }
        }
        n243 = Not(x=w378) -> (.not. x?=w381:bool)
        n244 = local read "Emt(T)/Enter(F)"() -> (w399:bool)
        n245 = And(x=w381, y=w400) -> (x .and. y?=w380:bool)
        n246 = Select(t="", s=w399, f="\n") -> (s? t:f=w398:string)
        n247 = Concatenate Strings(w392, w398) -> (w395:string)
        n248 = VISA Write(VISA resource name=w401, write buffer=w395) -> (VISA resource name out=w393:refnum<visa-resource-name>, error out=w394:errorcluster)  [unwired: 1 in, 1 out]
        n249 = flat-sequence {
          tunnel: w394 -> [w411]
          tunnel: [w411] -> w389
          tunnel: w393 -> [w410]
          tunnel: [w410] -> w390
          tunnel: u32 100 ("delay before read (ms)") -> [w412]
          frame #0 {
            n250 = Wait (ms)(milliseconds to wait=w412) -> ()  [unwired: 1 out]
          }
        }
        n251 = property class="Instr"(reference=w390, error in=w389) -> (reference out=w388:refnum<visa-resource-name>, error out=w386:errorcluster, "Serial Settings:Number of Bytes at Serial Port"=w387:u32)
        n252 = VISA Read(VISA resource name=w388, byte count=w387, error in (no error)=w386) -> (VISA resource name out=w402:refnum<visa-resource-name>, read buffer=w384:string)  [unwired: 2 out]
        n253 = call <vilib>:"Normalize End Of Line.vi"("end of line (Native)"=T3."UNIX", "string in"=w384) -> ("string out"=w379:string)  [unwired: 6 in]
        n254 = case shown="True" w380 {
          tunnel: w379 -> [_ w404]
          frame False {
          }
          frame True {
            n255 = String Subset(string=w404, length (rest)=1 ("length (rest)")) -> (substring=w407:string)  [unwired: 1 in]
            n256 = Equal?(x=w407, y="0") -> (x = y?=→"CPTE_0":bool)
            "CPTE =" <- w404
          }
        }
        n257 = local read "Log"() -> (w382:string)
        n258 = Concatenate Strings(w382, w379) -> (w383:string)
        n259 = local write "Log"(w383) -> ()
      }
    }
  }
  n260 = while {
    tunnel: w4 -> [_]
    tunnel: w5 -> [_]
    stop <- w424 stop-if-true
    w413 = "\n"
    w419 = 25 ("y")
    n261 = Search and Replace String(replace all?=TRUE ("replace all? (F)"), input string="Log", search string=w413, replace string=w413) -> (number of replacements=w421:i32)  [unwired: 4 in, 3 out]
    n262 = Increment(x=w421) -> (x+1=w420:i32)
    n263 = Greater?(x=w420, y=w419) -> (0:w417:bool)
    n264 = Subtract(x=w420, y=w419) -> (x-y=w416:i32)
    n265 = Select(t=w416, s=w417, f=0) -> (s? t:f=w418:i32)
    n266 = case shown="False" "Ручной(Т)/Авто" {
      tunnel: w418 -> [w426 _]
      frame False {
        n267 = property on="Log" class="Str"("Text.Scroll Position"=w426) -> ()  [unwired: 2 in, 2 out]
      }
      frame True {
      }
    }
    n268 = Wait (ms)(milliseconds to wait=u32 40) -> ()  [unwired: 1 out]
    n269 = local read "Стоп"() -> (w424:bool)
  }
  n270 = Close File(refnum=w12) -> ()  [unwired: 1 in, 2 out]
  n271 = call <instrlib>:"niDCPower Close.vi"("instrument handle"=w9) -> ()  [unwired: 10 in, 1 out]
  n272 = call <instrlib>:"niDCPower Close.vi"("instrument handle"=w8) -> ()  [unwired: 10 in, 1 out]
  n273 = call <instrlib>:"niDCPower Close.vi"("instrument handle"=w7) -> ()  [unwired: 10 in, 1 out]
  n274 = VISA Close(VISA resource name=w2) -> ()  [unwired: 1 in, 1 out]
